vi "ValvesFlow2019.vi"(6 "error in (no error)":errorcluster, 7 "Limite":dbl, 8 "ESTADO in":T2, 9 "Setpoints":T1 {"SP4" format="%.2f"; "SP3" format="%.2f"; "SP2" format="%.2f"; "SP1" format="%.2f"}) -> (0 "error out":errorcluster, 1 "ESTADO out":T2)   [LabVIEW 2013]
doc: "Use this template to create a dialog box. This template polls the state of the buttons on the front panel and does not use events. Use the Dialog Using Events template (not available in Base package) to create a dialog box with event handling."
uses:
  Controles/P2018 Arduino Control.ctl
  Controles/P2019 SetpointsFlows.ctl
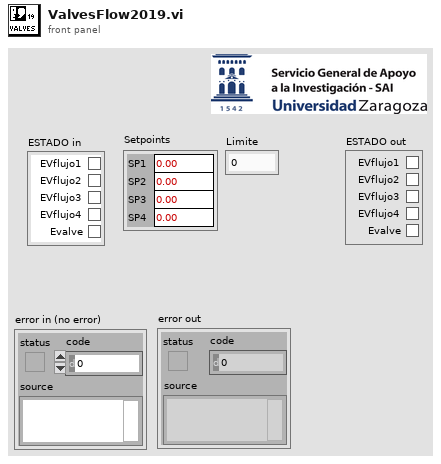
[diagram p1: front panel]
types:
  T1 = typedef "P2019 SetpointsFlows.ctl" = cluster{"SP1":dbl, "SP2":dbl, "SP3":dbl, "SP4":dbl}
  T2 = typedef "P2018 Arduino Control.ctl" = cluster{"EVflujo1":bool, "EVflujo2":bool, "EVflujo3":bool, "EVflujo4":bool, "Evalve":bool}
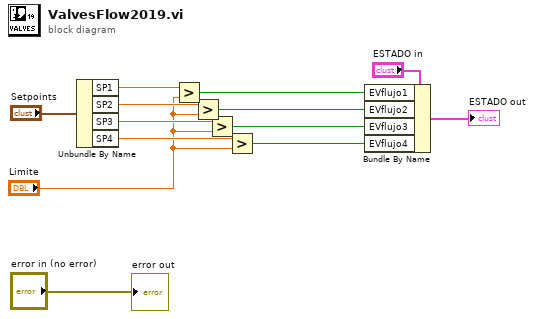
[diagram p0: block diagram]
diagram:
  n1 = Unbundle By Name("Setpoints") -> ("SP1"=w9:dbl, "SP2"=w8:dbl, "SP3"=w7:dbl, "SP4"=w6:dbl)
  n2 = Greater?(x=w9, y="Limite") -> (0:w2:bool)
  n3 = Greater?(x=w8, y="Limite") -> (0:w3:bool)
  n4 = Greater?(x=w7, y="Limite") -> (0:w4:bool)
  n5 = Greater?(x=w6, y="Limite") -> (0:w5:bool)
  n6 = Bundle By Name(cluster="ESTADO in", "EVflujo1"=w2, "EVflujo2"=w3, "EVflujo3"=w4, "EVflujo4"=w5) -> (→"ESTADO out":T2)
  "error out" <- "error in (no error)"
